vi "assign3Graphs.vi"(6 "wavegaph array in":refnum<vi>[](array[refnum]), 9 "All Channel in 2":waveform(dbl)[](array[waveform])=[{"t0"=timestamp(-8.331666700001072e-05 s since 1904-01-01), "dt"=1.6667e-08, "Y"=array[10000 elements]}, {"t0"=timestamp(-8.331666700001072e-05 s since 1904-01-01), "dt"=1.6667e-08, "Y"=array[10000 elements]}, {"t0"=timestamp(-8.331666700001072e-05 s since 1904-01-01), "dt"=1.6667e-08, "Y"=array[10000 elements]}], 10 "channel name Array":string[](array[string]), 11 "show3 array 2":refnum<vi>[](array[refnum])) -> ()   [LabVIEW 2013]
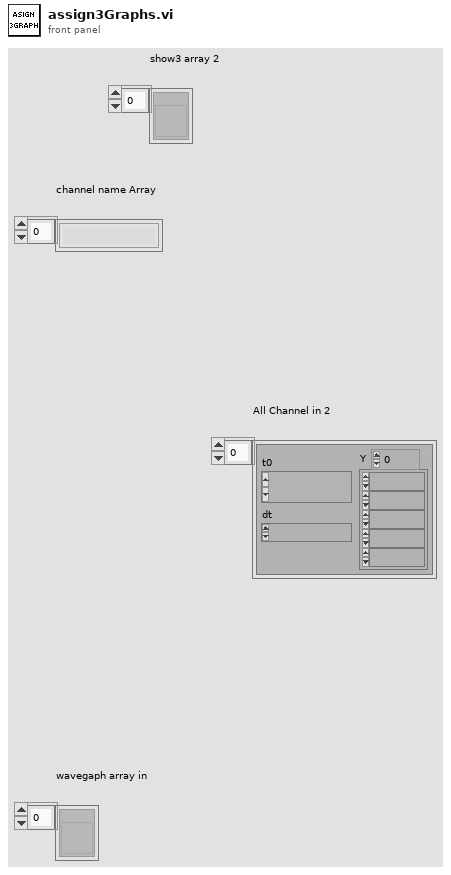
[diagram p1: front panel]
types:
  T1 = enum16{"Channel0", "Channel1", "Channel2", "Channel3", "Channel4", "Channel5", "Channel6", "Channel7"}
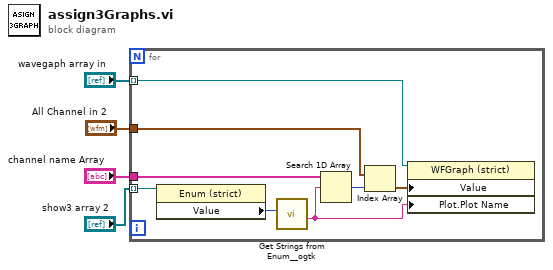
[diagram p0: block diagram]
diagram:
  n1 = for {
    tunnel: "show3 array 2" -> [w12] mode=indexing
    tunnel: "channel name Array" -> [w10]
    tunnel: "All Channel in 2" -> [w9]
    tunnel: "wavegaph array in" -> [w7] mode=indexing
    n2 = property class="Enum (strict)"(reference=w12) -> ("Value"=w11:T1)  [unwired: 1 in, 2 out]
    n3 = call <userlib>:"Get Strings from Enum__ogtk.vi"("Enum"=w11) -> ("String Value"=w5:string)  [unwired: 7 in, 3 out]
    n4 = Search 1D Array(1D array=w10, element=w5) -> (index of element=w8:i32)  [unwired: 1 in]
    n5 = Index Array(array=w9, index=w8) -> (element=w6:waveform(dbl))
    n6 = property class="WFGraph (strict)"(reference=w7, "Value"=w6, "Plot.Plot Name"=w5) -> ()  [unwired: 1 in, 2 out]
  }
